vi "Save Parsed Configuration.vi"(4 "HostToTarget DMAs":T2[](array[typedef]) {"Data Type" format="%.0x"}, 5 "Indicators":T4[](array[typedef]) {"Data Type" format="%.0x"}, 6 "TargetToHost DMAs":T2[](array[typedef]) {"Data Type" format="%.0x"}, 7 "Controls":T4[](array[typedef]) {"Data Type" format="%.0x"}, 8 "error in (no error)":errorcluster, 11 "Parent Ref in":T1 format="%.0x") -> (0 "error out":errorcluster, 3 "Section Ref out":T1 format="%.0x")   [LabVIEW 2020, in "FPGA Addon System Explorer.lvlib"]
uses:
  FPGA Addon System Explorer.lvlib
  Addon Shared/Types/Register Information.ctl
  Addon Shared/Types/FPGA Addon Data Type.ctl
  <vilib>/NI VeriStand/Custom Device API/Custom Device Item Ref.ctl
  Addon Shared/Types/DMA Information.ctl
  Addon Shared/Types/FG Action.ctl
  Addon Shared/SubVIs/Constants.vi
  <vilib>/NI VeriStand/Custom Device Tools/Custom Device Utility Library/NI VeriStand - Search for Item by GUID.vi
  <vilib>/NI/NI VeriStand Advanced SysDef API/SysDef API/SysDef.Property.Get.vi
  <vilib>/NI/NI VeriStand Advanced SysDef API/_SubVIs/SysDef.Property.Get.Variant.vi
  <vilib>/NI/NI VeriStand Advanced SysDef API/SysDef API/SysDef.Property.Set.vi
  <vilib>/NI/NI VeriStand Advanced SysDef API/_SubVIs/SysDef.Property.Set.Variant.vi
  <vilib>/NI VeriStand/Custom Device Tools/Custom Device Utility Library/Custom Device Utility Library.lvlib
  Addon Shared/FPGA Addon Shared.lvlib
  <vilib>/NI VeriStand/Custom Device API/Custom Device API.lvlib
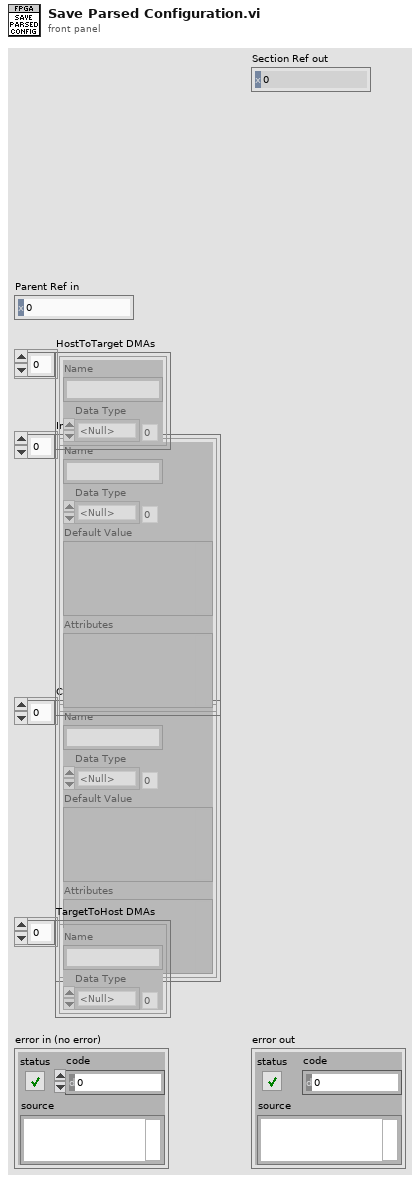
[diagram p1: front panel]
types:
  T1 = typedef "Custom Device API.lvlib/Custom Device Item Ref.ctl" = u64
  T2 = typedef "FPGA Addon Shared.lvlib/DMA Information.ctl" = cluster{"Name":string, "Data Type":T3}
  T3 = typedef "FPGA Addon Shared.lvlib/FPGA Addon Data Type.ctl" = enum8{"<Null>", "I8", "I16", "I32", "I64", "U8", "U16", "U32", "U64", "SGL", "Boolean", "Analog PWM In Settings", "Analog PWM In", "Digital PWM In Settings", "Digital PWM In", "Digital PWM Out", "Sine Out", "FXP", "FXP+/-24.5", "FXP+/-16.5", "FXP+/-32.8", "FXP+/-64.32", "FXP+/-16.7", "FXP+/-20.5", "FXP+/-27.5", "FXP+/-32.16", "FXP+16.3", "FXP+18.3", "Digital Static In", "Digital Static Out", "Digital Static In Settings", "Digital WSS Out", "Quad Encoder Settings", "Quad Encoder In", "Group"}
  T4 = typedef "FPGA Addon Shared.lvlib/Register Information.ctl" = cluster{"Name":string, "Data Type":T3, "Default Value":variant, "Attributes":variant}
  T5 = typedef "FPGA Addon Shared.lvlib/FG Action.ctl" = enum8{"GET", "SET"}
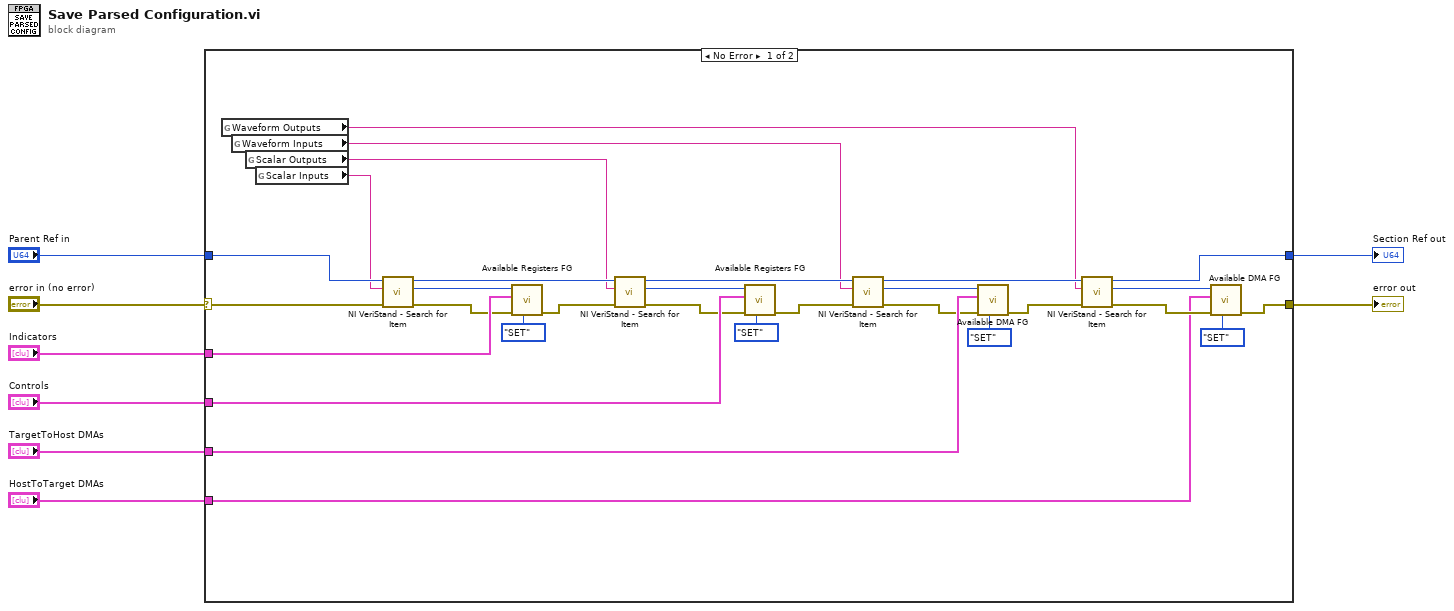
[diagram p0: block diagram]
diagram:
  n1 = case shown="No Error" "error in (no error)" {
    selector: "error in (no error)" -> [w9 w40]
    tunnel: "Controls" -> [w38 _]
    tunnel: "Indicators" -> [w37 _]
    tunnel: [w36 w39] -> w6
    tunnel: [w34 w40] -> w5
    tunnel: "HostToTarget DMAs" -> [w32 _]
    tunnel: "TargetToHost DMAs" -> [w27 _]
    tunnel: "Parent Ref in" -> [w14 w39]
    frame No Error {
      n2 = global read "Constants.vi" "Waveform Outputs"() -> (w10:string)
      n3 = global read "Constants.vi" "Waveform Inputs"() -> (w11:string)
      n4 = global read "Constants.vi" "Scalar Outputs"() -> (w12:string)
      n5 = global read "Constants.vi" "Scalar Inputs"() -> (w13:string)
      n6 = call-poly <vilib>:"NI VeriStand - Search for Item.vi"("error in"=w9, "Item GUID"=w13, "Section Ref in"=w14) -> ("error out"=w15:errorcluster, "Item Ref"=w16:T1, "Section Ref out"=w18:T1)  [unwired: 5 in, 1 out]
      n7 = call "Available Registers FG.vi"("Action"=FG_Action."SET", "error in (no error)"=w15, "Available Registers"=w37, "Item Ref"=w16) -> ("error out"=w17:errorcluster)  [unwired: 5 in, 2 out]
      n8 = call-poly <vilib>:"NI VeriStand - Search for Item.vi"("error in"=w17, "Item GUID"=w12, "Section Ref in"=w18) -> ("error out"=w23:errorcluster, "Item Ref"=w24:T1, "Section Ref out"=w20:T1)  [unwired: 5 in, 1 out]
      n9 = call "Available Registers FG.vi"("Action"=FG_Action."SET", "error in (no error)"=w23, "Available Registers"=w38, "Item Ref"=w24) -> ("error out"=w25:errorcluster)  [unwired: 5 in, 2 out]
      n10 = call-poly <vilib>:"NI VeriStand - Search for Item.vi"("error in"=w25, "Item GUID"=w11, "Section Ref in"=w20) -> ("error out"=w26:errorcluster, "Item Ref"=w19:T1, "Section Ref out"=w30:T1)  [unwired: 5 in, 1 out]
      n11 = call "Available DMA FG.vi"("Action"=FG_Action."SET", "error in (no error)"=w26, "Available DMA"=w27, "Item Ref"=w19) -> ("error out"=w29:errorcluster)  [unwired: 5 in, 2 out]
      n12 = call-poly <vilib>:"NI VeriStand - Search for Item.vi"("error in"=w29, "Item GUID"=w10, "Section Ref in"=w30) -> ("error out"=w33:errorcluster, "Item Ref"=w31:T1, "Section Ref out"=w36:T1)  [unwired: 5 in, 1 out]
      n13 = call "Available DMA FG.vi"("Action"=FG_Action."SET", "error in (no error)"=w33, "Available DMA"=w32, "Item Ref"=w31) -> ("error out"=w34:errorcluster)  [unwired: 5 in, 2 out]
    }
    frame Error {
    }
  }
  "Section Ref out" <- w6
  "error out" <- w5
